vi "waitForMotorToStop.vi"() -> ()   [LabVIEW 2020]
panel:
  out "newMotorPos":dbl
  out "motorPos":dbl
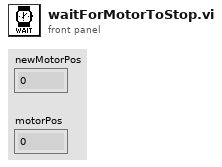
[diagram p1: front panel]
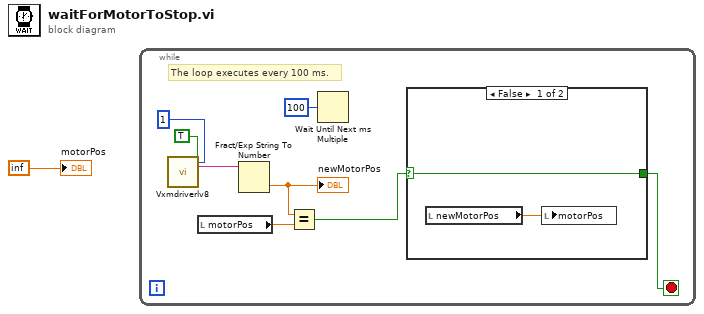
[diagram p0: block diagram]
diagram:
  n1 = while {
    stop <- w3 stop-if-true
    # "The loop executes every 100 ms."
    n2 = call "Vxmdriverlv8.Vi"("Get\nMotor\nPosition"=TRUE ("Get\nMotor\nPosition"), "Motor\nNumber"=1 ("Motor\nNumber")) -> ("Motor Position"=w7:string)  [unwired: 20 in, 5 out]
    n3 = local read "motorPos"() -> (w5:dbl)
    n4 = Fract/Exp String To Number(string=w7) -> (number=w6:dbl)  [unwired: 3 in, 1 out]
    "newMotorPos" <- w6
    n5 = Equal?(x=w6, y=w5) -> (x = y?=w4:bool)
    n6 = Wait Until Next ms Multiple(millisecond multiple=u32 100) -> ()  [unwired: 1 out]
    n7 = case shown="False" w4 {
      selector: w4 -> [w11 w12]
      tunnel: [w11 w12] -> w3
      frame False {
        n8 = local read "newMotorPos"() -> (w10:dbl)
        n9 = local write "motorPos"(w10) -> ()
      }
      frame True {
      }
    }
  }
  "motorPos" <- inf
